vi "test Get Attribute as DBL5.vi"(11 "Test Case In":refnum<class "Test Config From Excel Table.lvclass">) -> (0 "error out":errorcluster, 3 "Test Case Out":refnum<class "Test Config From Excel Table.lvclass">)   [LabVIEW 2020, in "Test Config From Excel Table.lvclass"]
uses:
  Test Config From Excel Table.lvclass
  C:/Program Files/National Instruments/LabVIEW 2025/vi.lib/Astemes/LUnit/Test Case.lvclass
  Source/Config from Excel Table/Config from Excel Table.lvclass
  <vilib>/Astemes/LUnit/Test Case.lvclass/Test Case.ctl
  Test Config From Excel Table.lvclass/Test Config From Excel Table.ctl
  <vilib>/Astemes/LUnit/Test Case.lvclass
  <vilib>/Peter/Open Xml/Source/Open Xml.lvlib
  4721e792-12f6-44ed-8f8f-b4c64d477831.vi
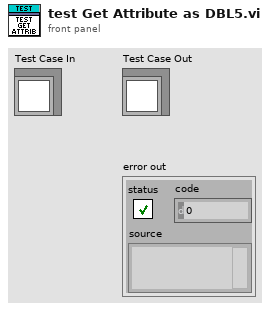
[diagram p1: front panel]
types:
  T1 = cluster{"Sheet Name":string, "Name":string, "Display Name":string, "Range or Cell Address":string}
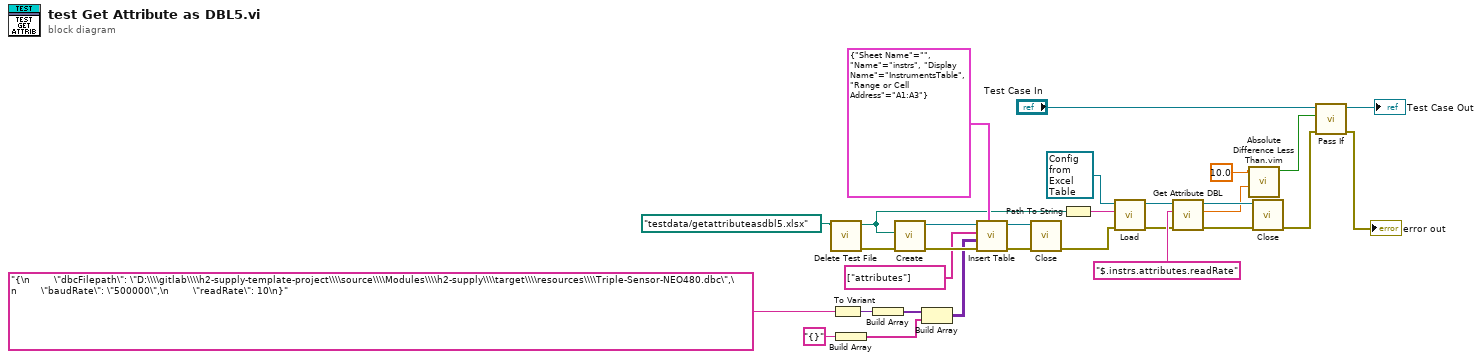
[diagram p0: block diagram]
diagram:
  n1 = call "Delete Test File.vi"("name or relative path"=path "testdata/getattributeasdbl5.xlsx") -> ("error out"=w19:errorcluster, "deleted path"=w7:path)  [unwired: 9 in]
  n2 = To Variant(anything="{\n        \"dbcFilepath\": \"D:\\\\gitlab\\\\h2-supply-template-project\\\\source\\\\Modules\\\\h2-supply\\\\target\\\\resources\\\\Triple-Sensor-NEO480.dbc\",\n        \"baudRate\": \"500000\",\n        \"readRate\": 10\n}") -> (Variant=w13:variant)
  n3 = Build Array("{}") -> (w4:string[])
  n4 = Build Array(w13) -> (w12:variant[])
  n5 = call <vilib>:"Create.vi"("error in"=w19, "Path"=w7) -> ("error out"=w18:errorcluster, "SpreadsheetDoc"=w10:refnum<k24>)  [unwired: 8 in]
  n6 = Build Array(w12, w4) -> (w11:variant[][])
  n7 = call <vilib>:"Insert Table.vi"("Location"=T1 {"Sheet Name"="", "Name"="instrs", "Display Name"="InstrumentsTable", "Range or Cell Address"="A1:A3"}, "error in"=w18, "Cell Values"=w11, "Header Names"=string[] ["attributes"], "SpreadsheetDoc in"=w10) -> ("error out"=w17:errorcluster, "SpreadsheetDoc out"=w8:refnum<k24>)  [unwired: 5 in]
  n8 = call <vilib>:"Close.vi"("error in"=w17, "SpreadsheetDoc"=w8) -> ("error out"=w9:errorcluster)  [unwired: 9 in]
  n9 = Path To String(path=w7) -> (string=w26:string)
  n10 = call-dynamic "Load.vi"("error in"=w9, "Source"=w26, "Config from Excel Table in"=refnum<class "Config from Excel Table.lvclass"> refnum ("Config from EXCEL Table.lvclass")) -> ("error out"=w20:errorcluster, "Config from Excel Table out"=w21:refnum<class "Config from Excel Table.lvclass">)  [unwired: 7 in]
  n11 = call-dynamic "Get Attribute DBL.vi"("error in"=w20, "Attribute"="$.instrs.attributes.readRate", "Config from Excel Table in"=w21) -> ("error out"=w23:errorcluster, "Value"=w1:dbl, "Config from Excel Table out"=w24:refnum<class "Config from Excel Table.lvclass">)  [unwired: 6 in]
  n12 = call "Absolute Difference Less Than.vim"("Number 2"=w1, "Number 1"=10.0 ("Value")) -> ("In Limit"=w2:bool)  [unwired: 9 in]
  n13 = call-dynamic <vilib>:"Close.vi"("error in"=w23, "Config from Excel Table in"=w24) -> ("error out"=w22:errorcluster)  [unwired: 8 in, 1 out]
  n14 = call <vilib>:"Pass If.vi"("error in (no error)"=w22, "Pass?"=w2, "LUnit Test Case In"="Test Case In") -> ("error out"=→"error out":errorcluster, "LUnit Test Case Out"=→"Test Case Out":refnum<class "Test Config From Excel Table.lvclass">)  [unwired: 7 in]
